vi "20170411-lecture3-3 stacked seq.vi"() -> ()   [LabVIEW 2014]
panel:
  out "x-y":u32
  out "Waveform Chart":dbl(graph)
  in  "Numeric":i32
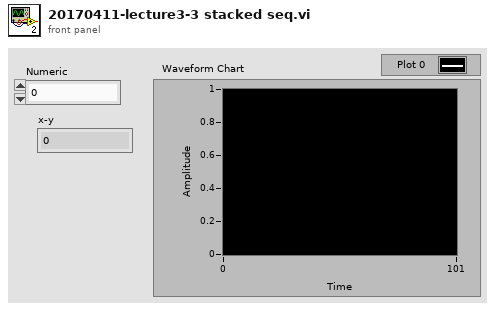
[diagram p1: front panel]
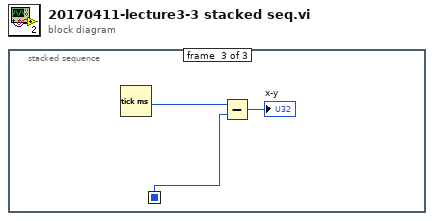
[diagram p0: block diagram]
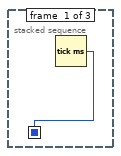
[diagram p2: hidden frame]
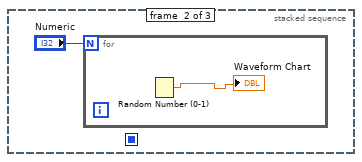
[diagram p3: hidden frame]
diagram:
  n1 = stacked-sequence {
    seq-local: [w1 _ _] -> [_ _ w4]
    frame #0 {
      n2 = Tick Count (ms)() -> (millisecond timer value=w1:u32)
    }
    frame #1 {
      n3 = for {
        N: "Numeric" -> [_]
        n4 = Random Number (0-1)() -> (number: 0 to 1=→"Waveform Chart":dbl)
      }
    }
    frame #2 {
      n5 = Tick Count (ms)() -> (millisecond timer value=w5:u32)
      n6 = Subtract(x=w5, y=w4) -> (x-y=→"x-y":u32)
    }
  }
